vi "MainPanel_20170525.vi"() -> (0 "ErrorOut":errorcluster)   [LabVIEW 2018] (continued)
-inf, -inf, -inf, -inf, -inf, -inf, -inf, -inf, -inf, -inf, -inf, -inf, -inf, -inf, -inf, -inf, -inf, -inf, -inf, -inf, -inf, -inf, -inf, -inf, -inf, -inf, -inf, -inf, -inf, -inf, -inf, -inf, -inf, -inf, -inf, -inf, -inf, -inf, -inf, -inf, -inf, -inf, -inf, -inf, -inf, -inf, -inf, -inf, -inf, -inf, -inf, -inf, -inf, -inf, -inf, -inf, -inf, -inf, -inf, -inf, -inf, -inf, -inf, -inf, -inf, -inf, -inf, -inf, -inf, -inf, -inf, -inf, -inf, -inf, -inf, -inf, -inf, -inf, -inf, -inf, -inf, -inf, -inf, -inf, -inf, -inf, -inf, -inf, -inf, -inf, -inf, -inf, -inf, -inf, -inf, -inf, -inf, -inf, -inf, -inf, -inf, -inf, -inf, -inf, -inf, -inf, -inf, -inf, -inf, -inf, -inf, -inf, -inf, -inf, -inf, -inf, -inf, -inf, -inf, -inf, -inf, -inf, -inf, -inf, -inf, -inf, -inf, -inf, -inf, -inf, -inf, -inf, -inf, -inf, -inf, -inf, -inf, -inf, -inf, -inf, -inf, -inf, -inf, -inf, -inf, -inf, -inf, -inf, -inf, -inf, -inf, -inf, -inf, -inf, -inf, -inf, -inf, -inf, -inf, -inf, -inf, -inf, -inf, -inf, -inf, -inf, -inf, -inf, -inf, -inf, -inf, -inf, -inf, -inf, -inf, -inf, -inf, -inf, -inf, -inf, -inf, -inf, -inf, -inf, -inf, -inf, -inf, -inf, -inf, -inf, -inf, -inf, -inf, -inf, -inf, -inf, -inf, -inf, -inf, -inf, -inf, -inf, -inf, -inf, -inf, -inf, -inf, -inf, -inf, -inf, -inf, -inf, -inf, -inf, -inf, -inf, -inf, -inf, -inf, -inf, -inf, -inf, -inf, -inf, -inf, -inf, -inf, -inf, -inf, -inf, -inf, -inf, -inf, -inf, -inf, -inf, -inf, -inf, -inf, -inf, -inf, -inf, -inf, -inf, -inf, -inf, -inf, -inf, -inf, -inf, -inf, -inf, -inf, -inf, -inf, -inf, -inf, -inf, -inf, -inf, -inf, -inf, -inf, -inf, -inf, -inf, -inf, -inf, -inf, -inf, -inf, -inf, -inf, -inf, -inf, -inf, -inf, -inf, -inf, -inf, -inf, -inf, -inf, -inf, -inf, -inf, -inf, -inf, -inf, -inf, -inf, -inf, -inf, -inf, -inf, -inf, -inf, -inf, -inf, -inf, -inf, -inf, -inf, -inf, -inf, -inf, -inf, -inf, -inf, -inf, -inf, -inf, -inf, -inf, -inf, -inf, -inf, -inf, -inf, -inf, -inf, -inf, -inf, -inf, -inf, -inf, -inf, -inf, -inf, -inf, -inf, -inf, -inf, -inf, -inf, -inf, -inf, -inf, -inf, -inf, -inf, -inf, -inf, -inf, -inf, -inf, -inf, -inf, -inf, -inf, -inf, -inf, -inf, -inf, -inf, -inf, -inf, -inf, -inf, -inf, -inf, -inf, -inf, -inf, -inf, -inf, -inf, -inf, -inf, -inf, -inf, -inf, -inf, -inf, -inf, -inf, -inf, -inf, -inf, -inf, -inf, -inf, -inf, -inf, -inf, -inf, -inf, -inf, -inf, -inf, -inf, -inf, -inf, -inf, -inf, -inf, -inf, -inf, -inf, -inf, -inf, -inf, -inf, -inf, -inf, -inf, -inf, -inf, -inf, -inf, -inf, -inf, -inf, -inf, -inf, -inf, -inf, -inf, -inf, -inf, -inf, -inf, -inf, -inf, -inf, -inf, -inf, -inf, -inf, -inf, -inf, -inf, -inf, -inf, -inf, -inf, -inf, -inf, -inf, -inf, -inf, -inf, -inf, -inf, -inf, -inf, -inf, -inf, -inf, -inf, -inf, -inf, -inf, -inf, -inf, -inf, -inf, -inf, -inf, -inf, -inf, -inf, -inf, -inf, -inf, -inf, -inf, -inf, -inf, -inf, -inf, -inf, -inf, -inf, -inf, -inf, -inf, -inf, -inf, -inf, -inf, -inf, -inf, -inf, -inf, -inf, -inf, -inf, -inf, -inf, -inf, -inf, -inf, -inf, -inf, -inf, -inf, -inf, -inf, -inf, -inf, -inf, -inf, -inf, -inf, -inf, -inf, -inf, -inf, -inf, -inf, -inf, -inf, -inf, -inf, -inf, -inf, -inf, -inf, -inf, -inf, -inf, -inf, -inf, -inf, -inf, -inf, -inf, -inf, -inf, -inf, -inf, -inf, -inf, -inf, -inf, -inf, -inf, -inf, -inf, -inf, -inf, -inf, -inf, -inf, -inf, -inf, -inf, -inf, -inf, -inf, -inf, -inf, -inf, -inf, -inf, -inf, -inf, -inf, -inf, -inf, -inf, -inf, -inf, -inf, -inf, -inf, -inf, -inf, -inf, -inf, -inf, -inf, -inf, -inf, -inf, -inf, -inf, -inf, -inf, -inf, -inf, -inf, -inf, -inf, -inf, -inf, -inf, -inf, -inf, -inf, -inf, -inf, -inf, -inf, -inf, -inf, -inf, -inf, -inf, -inf, -inf, -inf, -inf, -inf, -inf, -inf, -inf, -inf, -inf, -inf, -inf, -inf, -inf, -inf, -inf, -inf, -inf, -inf, -inf, -inf, -inf, -inf, -inf, -inf, -inf, -inf, -inf, -inf, -inf, -inf, -inf, -inf, -inf, -inf, -inf, -inf, -inf, -inf, -inf, -inf, -inf, -inf, -inf, -inf, -inf, -inf, -inf, -inf, -inf, -inf, -inf, -inf, -inf, -inf, -inf, -inf, -inf, -inf, -inf, -inf, -inf, -inf, -inf, -inf, -inf, -inf, -inf, -inf, -inf, -inf, -inf, -inf, -inf, -inf, -inf, -inf, -inf, -inf, -inf, -inf, -inf, -inf, -inf, -inf, -inf, -inf, -inf, -inf, -inf, -inf, -inf, -inf, -inf, -inf, -inf, -inf, -inf, -inf, -inf, -inf, -inf, -inf, -inf, -inf, -inf, -inf, -inf, -inf, -inf, -inf, -inf, -inf, -inf, -inf, -inf, -inf, -inf, -inf, -inf, -inf, -inf, -inf, -inf, -inf, -inf, -inf, -inf, -inf, -inf, -inf, -inf, -inf, -inf, -inf, -inf, -inf, -inf, -inf, -inf, -inf, -inf, -inf, -inf, -inf, -inf, -inf, -inf, -inf, -inf, -inf, -inf, -inf, -inf, -inf, -inf, -inf, -inf, -inf, -inf, -inf, -inf, -inf, -inf, -inf, -inf, -inf, -inf]
  out "df (Hz)":dbl=15258.7890625
  in  "AutoScale Y Noise":bool caption="AutoScale Y"
  in  "AvgAvg":bool caption="Average over 1 minute"
  out "Freq History 72 Co":cluster{dbl, dbl, dbl}(graph)
  out "Freq History 84 Co":cluster{dbl, dbl, dbl}(graph)
  out "84CoCalFrq":dbl format="%#.9f"
  out "MaxValue_Cal_84X":dbl format="%#.2g"
  out "84CoBeacFrq":dbl format="%#.9f"
  out "MaxValue_Cal_72X":dbl format="%#.2g"
  out "72CoCalFrq":dbl format="%#.9f"
  out "72CoBeacFrq":dbl format="%#.2f"
  out "ADAM-Noise":dbl format="%#.2g"
  out "ADAM-CalEncl":dbl format="%#.2g"
  out "ADAM-XPol":dbl format="%#.2g"
  out "ADAM-Co":dbl format="%#.2g"
  out "TE_Front":dbl format="%#.2g"
  out "TE_Bottom":dbl format="%#.2g"
  out "TE_Air":dbl format="%#.2g"
  out "InclEl":dbl format="%#.2g"
  out "InclAz":dbl format="%#.2g"
  out "MaxValue_Cal_84Co":dbl format="%#.2g"
  out "MaxValue_Cal_72Co":dbl format="%#.2g"
  out "+28":dbl format="%#.2g"
  out "+15":dbl format="%#.2g"
  out "+12":dbl format="%#.2g"
  out "+6":dbl format="%#.2g"
  out "+5":dbl format="%#.2g"
  out "-5V":dbl format="%#.2g"
  out "ConnextIntTemp":dbl format="%#.2g"
  in  "AlarmThresholds_OneChan":T12={"Enbl"=FALSE, "ErrsAndWarns"={2.256637168141593, 5.663716814159292, 7.168141592920354, 9.336283185840708}} {"ErrsAndWarns" scale=0.0..10.0}
  in  "AlarmSettings":T13={"TC13"={"Enbl"=FALSE, "ErrsAndWarns"={0.0, 5.663716814159292, 7.168141592920354, 8.584070796460177}}, "AI1"={"Enbl"=FALSE, "ErrsAndWarns"={0.0, 5.663716814159292, 7.168141592920354, 8.584070796460177}}, "AI2"={"Enbl"=FALSE, "ErrsAndWarns"={0.0, 5.663716814159292, 7.168141592920354, 8.584070796460177}}, "AI3"={"Enbl"=FALSE, "ErrsAndWarns"={0.0, 5.663716814159292, 7.168141592920354, 8.584070796460177}}, "AI4"={"Enbl"=FALSE, "ErrsAndWarns"={0.0, 5.663716814159292, 7.168141592920354, 8.584070796460177}}, "AI5"={"Enbl"=FALSE, "ErrsAndWarns"={0.0, 5.663716814159292, 7.168141592920354, 8.584070796460177}}, "AI6"={"Enbl"=FALSE, "ErrsAndWarns"={0.0, 5.663716814159292, 7.168141592920354, 8.584070796460177}}, "AI18"={"Enbl"=FALSE, "ErrsAndWarns"={0.0, 5.663716814159292, 7.168141592920354, 8.584070796460177}}, "AI19"={"Enbl"=FALSE, "ErrsAndWarns"={0.0, 5.663716814159292, 7.168141592920354, 8.584070796460177}}, "TE1"={"Enbl"=FALSE, "ErrsAndWarns"={0.0, 5.663716814159292, 7.168141592920354, 8.584070796460177}}, "TE2"={"Enbl"=TRUE, "ErrsAndWarns"={0.0, 5.663716814159292, 7.168141592920354, 8.584070796460177}}, "TE3"={"Enbl"=FALSE, "ErrsAndWarns"={0.0, 5.663716814159292, 7.168141592920354, 8.584070796460177}}, "ADAM1"={"Enbl"=FALSE, "ErrsAndWarns"={0.0, 5.663716814159292, 7.168141592920354, 8.584070796460177}}, "ADAM2"={"Enbl"=FALSE, "ErrsAndWarns"={0.0, 5.663716814159292, 7.168141592920354, 8.584070796460177}}, "ADAM3"={"Enbl"=FALSE, "ErrsAndWarns"={0.0, 5.663716814159292, 7.168141592920354, 8.584070796460177}}, "ADAM4"={"Enbl"=FALSE, "ErrsAndWarns"={0.0, 5.663716814159292, 7.168141592920354, 8.584070796460177}}, "72CoBeacFreq"={"Enbl"=FALSE, "ErrsAndWarns"={0.0, 5.663716814159292, 7.168141592920354, 8.584070796460177}}, "72CoCalFreq"={"Enbl"=FALSE, "ErrsAndWarns"={0.0, 5.663716814159292, 7.168141592920354, 8.584070796460177}}, "84CoBeacFreq"={"Enbl"=FALSE, "ErrsAndWarns"={0.0, 5.663716814159292, 7.168141592920354, 8.584070796460177}}, "84CoCalFreq"={"Enbl"=FALSE, "ErrsAndWarns"={0.0, 5.663716814159292, 7.168141592920354, 8.584070796460177}}, "72Co_CalTonePwr"={"Enbl"=FALSE, "ErrsAndWarns"={-110.0, -90.0, -65.0, -60.0}}, "72X_CalTonePwr"={"Enbl"=FALSE, "ErrsAndWarns"={0.0, 5.663716814159292, 7.168141592920354, 8.584070796460177}}, "84Co_CalTonePwr"={"Enbl"=FALSE, "ErrsAndWarns"={0.0, 5.663716814159292, 7.168141592920354, 8.584070796460177}}, "84X_CalTonePwr"={"Enbl"=FALSE, "ErrsAndWarns"={0.0, 5.663716814159292, 7.168141592920354, 8.584070796460177}}} {"84X_CalTonePwr"."ErrsAndWarns" scale=-120.0..-45.0; "72X_CalTonePwr"."ErrsAndWarns" scale=-120.0..-45.0; "84Co_CalTonePwr"."ErrsAndWarns" scale=-120.0..-45.0; "72Co_CalTonePwr"."ErrsAndWarns" scale=-120.0..-45.0; "84CoCalFreq"."ErrsAndWarns" scale=24.9..25.1; "84CoBeacFreq"."ErrsAndWarns" scale=25.5..27.0; "72CoCalFreq"."ErrsAndWarns" scale=24.9..25.1; "72CoBeacFreq"."ErrsAndWarns" scale=25.5..27.0; "ADAM4"."ErrsAndWarns" scale=30.0..52.0; "ADAM3"."ErrsAndWarns" scale=30.0..52.0; "ADAM2"."ErrsAndWarns" scale=30.0..52.0; "ADAM1"."ErrsAndWarns" scale=30.0..52.0; "TE3"."ErrsAndWarns" scale=30.0..52.0; "TE2"."ErrsAndWarns" scale=30.0..52.0; "TE1"."ErrsAndWarns" scale=20.0..52.0; "AI19"."ErrsAndWarns" scale=0.0..60.0; "AI18"."ErrsAndWarns" scale=-10.0..10.0; "AI6"."ErrsAndWarns" scale=0.0..35.0; "AI5"."ErrsAndWarns" scale=0.0..20.0; "AI4"."ErrsAndWarns" scale=0.0..15.0; "AI3"."ErrsAndWarns" scale=0.0..10.0; "AI2"."ErrsAndWarns" scale=0.0..10.0; "TC13"."ErrsAndWarns" scale=-10.0..40.0}
  out "Elapsed_SNR_Timer":dbl caption="Elapsed SNR Timer"
  out "BlowerPower":dbl format="%#.2g"
  out "GeneratorExhaust":dbl format="%#.2g"
  in  "Trouble Shooting Tabs":T14(tab)
  out "Q Probes":T15
  out "Probe 21":fxp<+/-,24,5>=-4.57763671875e-05
  out "Probe 22":fxp<+/-,54,35>=-15871.999969482422
  out "Probe 23":fxp<+/-,54,1>=-7.629394517039145e-06
  out "Probe 24":fxp<+/-,16,1>
  out "I Probes":T15
  out "Probe 3":fxp<+/-,39,24>=-0.003662109375
  out "Probe 1":i16=-27
  out "Probe 2":fxp<+/-,16,16>
  out "Probe 5":fxp<+/-,16,2>
  out "Probe 7":fxp<+/-,18,1>
  out "Probe Offsetd":fxp<+/-,16,16>
  in  "Target to Probe":T16=enum."4"
  in  "Time Domain Tabs":enum32{"72 Co", "72 X", "84 Co", "84 X"}(tab)
  out "TimeDomainCal 72Co":ext[](graph)
  out "TimeDomainBeac 72Co":ext[](graph)
  out "TimeDomainCal 72 X":ext[](graph)
  out "TimeDomainBeacon 72 X":ext[](graph)
  out "TimeDomainCal 84 Co":ext[](graph)
  out "TimeDomain Beac 84 Co":ext[](graph)
  out "TimeDomainCal 84 X":ext[](graph)
  out "TimeDomainBeacon 84 X":ext[](graph)
  out "Memory Used":dbl(graph)=797012.0
  out "CalShift 2":dbl=24999500.0 format="%#_10g"
  out "BeaconShift 2":dbl=26246000.0 format="%#_10g"
  out "BeaconShift":dbl=26246000.0 format="%#_10g"
  out "CalShift":dbl=24999500.0 format="%#_10g"
  out "Memory Used By LV (KB)":dbl=797012.0
  out "BeaconShift 4":dbl=26244800.0 format="%#_10g"
  out "BeaconShift 3":dbl=26246000.0 format="%#_10g"
  out "CalShift 3":dbl=24999500.0 format="%#_10g"
  out "CalShift 4":dbl=24998000.0 format="%#_10g"
  in  "MemoryPlotRate":dbl=30.0 format="%#_13g"
  out "SPVSR_Count":i32
  out "SPVSR_Queue":i32
  out "FP_Count":i32
  out "# in FP queue":i32
  out "Digitizer 1 Init Attempts":i32
  out "Digitizer 2 Init Attempts":i32
  in  "noise_ctrl":bool
  in  "72GHz_ctrl":bool=TRUE
  in  "84GHz_ctrl":bool=TRUE
  in  "base path":path=path "C:/ConnexTest" caption="Local Storage path for data logs"
  in  "NAS path":path=path "C:/ConnexData"
  in  "ThreshFile":path=path "C:/Users/bruce wayne/Desktop/ATA_Source_20180912/thresholds.csv" caption="Thresholds file"
  in  "Exit":bool
  in  "Stop":bool
  # "Ver 20220331"
  # "Low pass filter applied to chart.\nTo turn filter off, set New Value Weighting to 1."
  # "Angle_out = [(V_reading – Vmin) / Vmax ) * (Angle_max - Angle_min) + Angle_min + Angle_offset ] * (-1 if pos_neg toggle switch is on)\n\nThe default (equivalent to current equation) values would be\nVmin = 0\nVmax = 4.5\nAngle_min = -90\nAngle_range = Angle_max-Angle_min\nAngle_max = 90\nAngle_offset = 0\nPos_neg = off"
  # "v 2022_03_08"
  # "72 Cross Tracking Frequency is linked to 72 Co"
  # "84 Cross Tracking Frequency is linked to 84 Co"
  # "72 GHz"
  # "84 GHz"
  # "Do not use \"Tab\" to commit values. Use \"Enter\" or click off of the control."
  # "Enable/disable"
  # "The digital readouts display the same errors and \nwarnings with more precision."
  # "Low Error"
  # "Low Warning"
  # "High Warning"
  # "High Error"
  # "seconds"
  # "Copyright © 2022 Epimedia, Inc. All Rights Reserved.\n\nThe Epimedia Application Library is Copyright © 2009-2022 Epimedia, Inc. \nAll Rights Reserved. Used under license."
  # "I Probes"
  # "Q Probes"
  # "-1 to 0.999, d:7.629e-6"
  # "Shifted"
  # "I16"
  # "-1 to 1, d:1.92e-7"
  # "From digitizer"
  # "Filtered Step 4"
  # "-3.27e4 to 3.27e4, d:1"
  # "-1 to 1, d:1.92e-7"
  # "To FXP"
  # "Scaled and reduced data size"
  # "-3.27e4 to 3.27e4, d:1"
  # "-1 to 1, d:1.92e-7"
  # "Filtered Step 5"
  # "-6.55e4 to 6.55e4, d:3.05e-5"
  # "-8.39e6 to 8.39e6, d:1.19e-7"
  # "Scaled"
  # "Scaled after Step 5"
  # "XXX"
  # "-2 to 2, d:2.38e-7"
  # "-2 to 1.999, d:6.10e-5"
  # "Filtered Step 6"
  # "Filtered stage A"
  # "-1.677e7 to 1.677e7, d:2.38e-7"
  # "Scaled after Step 6"
  # "XXX"
  # "-2.62e5 to 2.62e5, d:6.10e-5"
  # "Scaled (Step 1 Scale)"
  # "-1 to 1, d:1.82e-12"
  # "Filtered Step 7"
  # "-8.39e6 to 8.39e6, d:1.82e-12"
  # "Filtered after Step 7"
  # "XXX"
  # "-8.39e6 to 8.39e6, d:1.82e-12"
  # "Sent to host\nIdentical to 18"
  # "Noise Floor"
  # "-4 to 4"
  # "-3.35e7 to 3.35e7, d:4.7e-7"
  # "-1 to 1, d:1.4e-14"
  # "-1 to .99, d:3.05e-5"
  # "The following shift variables are used to scale\nthe x-axis of the plots on the the Spectrum tab"
  # "The noise source has been disconnected. Please see technical manual for further information."
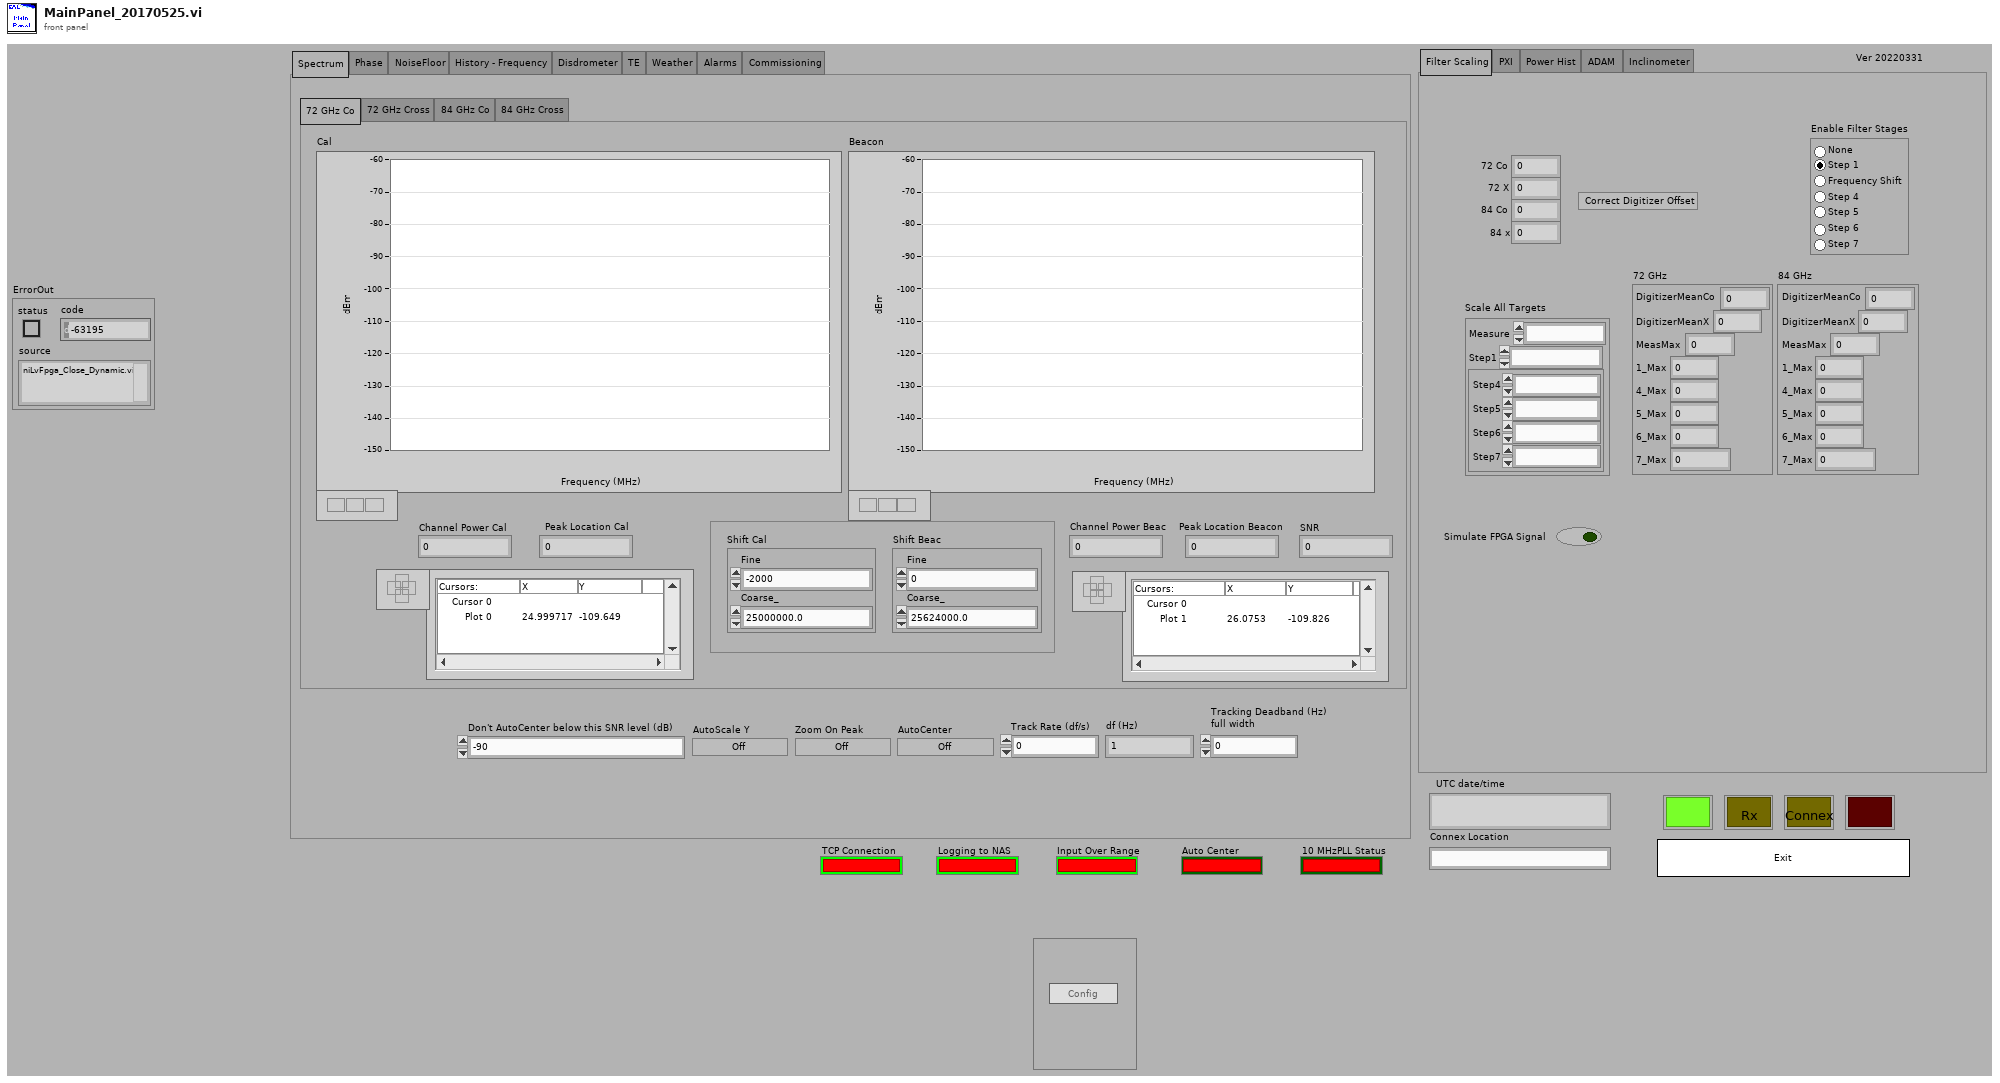
[diagram p1: front panel]
types:
  T1 = enum32{"Filter Scaling", "PXI", "Power Hist", "ADAM", "Inclinometer"}
  T2 = typedef "SaturationMonitor.ctl" = cluster{"MeasMean0":dbl, "MeasMean1":dbl, "MeasMax":dbl, "1_Max":dbl, "4_Max":dbl, "5_Max":dbl, "6_Max":dbl, "7_Max":dbl}
  T3 = typedef "ScaleTargetClust.ctl" = cluster{"Measure":fxp<+/-,16,1>, "Step1":fxp<+/-,17,17>, "Scale":T4}
  T4 = typedef "FPGA_Scale.ctl" = cluster{"Step4":fxp<+/-,23,23>, "Step5":fxp<+/-,23,23>, "Step6":fxp<+/-,23,23>, "Step7":fxp<+/-,23,23>}
  T5 = typedef "FilterEnableRadio.ctl" = enum32{"None", "Step 1", "Frequency Shift", "Step 4", "Step 5", "Step 6", "Step 7"}
  T6 = cluster{"Cal Smooth":dbl, "Beac Smooth":dbl, "Cal Smooth":dbl, "Beac Smooth":dbl, "Cal Smooth":dbl, "Beac Smooth":dbl, "Cal Smooth":dbl, "Beac Smooth":dbl}
  T7 = typedef "Inclinometer_User_Cfg.ctl" = cluster{"Vmin":dbl, "Vmax":dbl, "Angle_min":dbl, "Angle_max":dbl, "Offset":dbl, "Pos_Neg":bool}
  T8 = cluster{"Ai18_InclinometerAz":dbl, "Ai19_InclinometerEl":dbl}
  T9 = enum32{"Spectrum", "Phase", "NoiseFloor", "History - Frequency", "Disdrometer", "TE", "Weather", "Alarms", "Commissioning"}
  T10 = enum32{"72 GHz Co", "72 GHz Cross", "84 GHz Co", "84 GHz Cross"}
  T11 = typedef "FreqShift.ctl" = cluster{"Fine":dbl, "Coarse_":dbl}
  T12 = typedef "AlarmThresh_OneChan.ctl" = cluster{"Enbl":bool, "ErrsAndWarns":cluster{dbl, dbl, dbl, dbl}}
  T13 = typedef "AlarmSettingsClust.ctl" = cluster{"TC13":T12, "AI1":T12, "AI2":T12, "AI3":T12, "AI4":T12, "AI5":T12, "AI6":T12, "AI18":T12, "AI19":T12, "TE1":T12, "TE2":T12, "TE3":T12, "ADAM1":T12, "ADAM2":T12, "ADAM3":T12, "ADAM4":T12, "72CoBeacFreq":T12, "72CoCalFreq":T12, "84CoBeacFreq":T12, "84CoCalFreq":T12, "72Co_CalTonePwr":T12, "72X_CalTonePwr":T12, "84Co_CalTonePwr":T12, "84X_CalTonePwr":T12}
  T14 = enum32{"FPGA Probes", "Time Domain", "Win Probes", "Cal Tone Controls", "Paths"}
  T15 = cluster{"Probe 8":fxp<+/-,18,1>, "Probe 9":fxp<+/-,24,1>, "Probe 10":fxp<+/-,24,1>, "Probe 11":fxp<+/-,24,1>, "Probe 12":fxp<+/-,47,24>, "Probe 13":fxp<+/-,24,1>, "Probe 14":fxp<+/-,25,2>, "Probe 15":fxp<+/-,48,25>, "Probe 16":fxp<+/-,24,1>, "Probe 17":fxp<+/-,25,2>, "Probe 18":fxp<+/-,48,25>, "Probe 19":fxp<+/-,24,1>, "Probe20":fxp<+/-,24,1>}
  T16 = typedef "TargetNumber.ctl" = enum16{"1", "2", "3", "4"}
  T17 = typedef "LogLoopEnum.ctl" = enum16{"Log_Init", "Log_Config", "Log_CfgAlarm", "Log_TimeDomain", "Log_Tone", "Log_NoiseTrace", "Log_NoiseSum", "Log_DO", "Log_AI", "Log_TC", "Log_Disdrom", "Log_Weather", "Log_TE", "Log_ADAM", "Log_UPS", "Log_ChkTime", "Log_Alarm", "Log_SSH", "Log_Write", "Log_Exit"}
  T18 = typedef "TCP_Loop.ctl" = enum16{"TCP_Write", "TCP_ChkTime", "TCP_Exit"}
  T19 = typedef "10Hz_Loop_Enum.ctl" = enum16{"10Hz_Init", "10Hz_Cfg", "10Hz_NewData", "10Hz_Write", "10Hz_Stop"}
  T20 = typedef "FP_Loop_Clust.ctl" = cluster{"Alarms":T21, "Spectrum 1":dbl[], "Spectrum 2":dbl[], "Spectrum 3":dbl[], "Spectrum 4":dbl[], "HistoryWeighting":dbl, "NoiseFloorSums":T22, "PwrHist":T23}
  T21 = typedef "DigOutClust.ctl" = cluster{"Green":bool, "Rx_Yell":bool, "Cx_Yell":bool, "Red":bool, "Source":string}
  T22 = typedef "NoiseFLoorSums.ctl" = cluster{"1":dbl, "2":dbl, "3":dbl, "4":dbl}
  T23 = typedef "PowerHistory_All.ctl" = cluster{"72Co":cluster{"Cal":dbl, "Cal Smooth":dbl, "Beac":dbl, "Beac Smooth":dbl, "NoiseFloorSum":dbl, "NoiseFloorSum Smooth":dbl}, "72X":cluster{"Cal":dbl, "Cal Smooth":dbl, "Beac":dbl, "Beac Smooth":dbl, "NoiseFloorSum":dbl, "NoiseFloorSum Smooth":dbl}, "84Co":cluster{"Cal":dbl, "Cal Smooth":dbl, "Beac":dbl, "Beac Smooth":dbl, "NoiseFloorSum":dbl, "NoiseFloorSum Smooth":dbl}, "84X":cluster{"Cal":dbl, "Cal Smooth":dbl, "Beac":dbl, "Beac Smooth":dbl, "NoiseFloorSum":dbl, "NoiseFloorSum Smooth":dbl}}
  T24 = typedef "AI_Type_Enum.ctl" = enum16{"AI", "TC"}
  T25 = typedef "HWQueueElements.ctl" = enum16{"HW_Init", "HW_UpdtCfg", "HW_Start", "HW_Pause", "HW_Run", "HW_Cls", "HW_Exit"}
  T26 = typedef "FP_Loop_Enum.ctl" = enum16{"FP_Init", "FP_Scale", "FP_Tone", "FP_Noise", "FP_Probes", "FP_PXI", "FP_AI", "FP_TC", "FP_PWR_Hist", "FP_Alarm", "FP_Exit"}
  T27 = typedef "DigiLoopEnum.ctl" = enum16{"Dig_Init", "Digi_Write", "Digi_Exit"}
  T28 = typedef "NoiseQueueElements.ctl" = enum16{"Noise_Startup", "Noise_Init", "Noise_Macro", "Noise_Config", "Noise_NewData", "Noise_Transform", "Noise_SumdTrace", "Noise_Send", "Noise_Probes", "Noise_Exit"}
  T29 = typedef "MasterCluster.ctl" = cluster{"Admin":T30, "RTConfig":T32, "SMS":T33, "FPGA":T34, "Config":T35, "Stat":T41, "Alarm":T13}
  T30 = typedef "AdminCluster.ctl" = cluster{"Lvl":T31, "Pwd":string}
  T31 = typedef "UserLevelEnum.ctl" = enum16{"Admin", "Operator"}
  T32 = typedef "RT_Config.ctl" = cluster{"Arm":bool, "Number":dbl, "String":string}
  T33 = typedef "SMSDataCluster.ctl" = cluster{"Enbl?":bool, "Addr":string[]}
  T34 = typedef "FPGA_Config_Clust.ctl" = cluster{"Target":T16, "Channel":T16, "Ref1":refnum<k20>, "Ref2":refnum<k20>}
  T35 = typedef "Config_Clust.ctl" = cluster{"UsrCfg":T36, "FP_User":T38}
  T36 = typedef "UserConfig.ctl" = cluster{"Paths":T37, "SampleRate":dbl}
  T37 = typedef "PathsCluster.ctl" = cluster{"CfgFile":path, "LogFolder":path, "LogFile":path, "NAS path":path, "ThreshFile":path, "RedunFolder":path}
  T38 = typedef "FrontPanel_UserConfig.ctl" = cluster{"#NoiseSums":u32, "Max_df":u32, "AvgAvg":bool, "#Avg":u16, "AutoCenter":bool, "Inclin":T7, "1":T39, "2":T39, "3":T39, "4":T39, "Target to Probe":T16, "SNR_Thresh":dbl, "Paths":T37, "Connex_Location":string, "SimulateFPGA":bool, "Deadband":dbl}
  T39 = typedef "FP_UserTargetConfig.ctl" = cluster{"Cal_":T11, "Beac":T11, "Scale":T4, "Offset":fxp<+/-,16,16>, "Scale_Noise":fxp<+/-,30,30>, "Scale_Step1":fxp<+/-,17,17>, "Scale_In_RT":ext, "ScaleMeas":fxp<+/-,16,1>, "FreqsToRemove":i32[], "Width":i32[], "ScaleMeasEnum":T40, "FilterEnab":T5}
  T40 = typedef "ScaleMeasure.ctl" = enum16{"1", "10", "50", "42"}
  T41 = typedef "SystemStatusCluster.ctl" = cluster{"SysState":T42, "TrackRate":bool, "AutoCentr":bool}
  T42 = typedef "SystemStateEnum.ctl" = enum16{"Init", "Idle", "Running", "System Fault", "System Error", "Exit"}
  T43 = typedef "DataQueueElements.ctl" = enum16{"Data_Init", "Data_Config", "Data_AddData", "Data_FreqShift", "Data_FPGA_Write", "Data_Transform", "Data_Send", "Data_Exit"}
  T44 = typedef "MainQueueElements.ctl" = enum16{"Spvsr_InitQ", "Spvsr_RfrshPnl", "Spvsr_InitSW", "Spvsr_InitCtrls", "Spvsr_Cursors", "Spvsr_StrtHWLp", "Spvsr_Stop", "Spvsr_NewData", "Spvsr_ScaleGraphs", "Spvsr_Error", "Spvsr_About", "Spvsr_Config", "Spvsr_FPConfig", "Spvsr_AlarmCfg", "Spvsr_DigitzOffs", "FP_AO_ctrl", "Spvsr_RestartWarn", "Spvsr_AutoCenter", "Spvsr_TrackRate", "Spvsr_ChkTime", "Spvsr_Admin", "Spvsr_Exit"}
  T45 = typedef "HDF5_10HzRefs.ctl" = cluster{"72Co_dset":T46, "84Co_dset":T46, "FileRef":T46}
  T46 = typedef "hid_t.ctl" = i32
  T47 = typedef "WatchdogTimer_Enum.ctl" = enum16{"ResetAll", "CheckAll", "HW1", "HW2", "Tones", "FP", "Noise", "Log", "TCP", "AI", "TC", "ADAM", "Disdrom", "TE", "Weather"}
  T48 = enum8{"Enabled", "Disabled", "Disabled and Grayed Out"}
  T49 = typedef "AI_Loop_Enum.ctl" = enum16{"AI_Init", "AI_Config", "AI_Alarm", "AI_Read", "AI_ChkTime", "AI_Exit"}
  T50 = typedef "LVCursorListTypeDef.ctl" = cluster{"Name":string, "Color":u32, "Style":u8, "Point Style":u8, "Name Visible":bool, "Allow Drag":bool, "Cursor Mode":u32, "Plot":i32, "Index":i32, "Position":cluster{"X":dbl, "Y":dbl}, "X Scale":u32, "Y Scale":u32, "Watch Plots":i32[], "Watch All Plots":bool, "Plot Area":i32, "Label Offset":cluster{"X":dbl, "Y":dbl}}[]
  T51 = typedef "AO_Loop_Enum.ctl" = enum16{"AO_Init", "AO_Write", "AO_Exit"}
  T52 = typedef "TargetToneData.ctl" = cluster{"Cal":T53, "Beac":T53, "Time":timestamp[], "Saturat":T2}
  T53 = typedef "ChannelToneData.ctl" = cluster{"Shift_":dbl, "Peak_ToFPGA":dbl, "MaxValue":dbl, "MaxIndex":i32, "Tone":T54, "TimeDomainI":ext[], "TimeDomainQ":ext[], "PwrSpectrum":dbl[], "RunningAvgFreq":dbl, "ISpectPos":dbl[], "ISpectNeg":dbl[], "QSpectPos":dbl[], "QSpectNeg":dbl[], "10Hz_PwrSpectr":dbl[][], "SNR":dbl, "AliasWarn":bool, "10Hz_Peak":dbl[], "ISpect+-":dbl[], "QSpect+-":dbl[], "TimeStamp":timestamp, "I_Index":ext[], "Q_Index":ext[], "10MHz":bool}
  T54 = typedef "ToneInfoClust.ctl" = cluster{"PkLocTrak":dbl, "PkLocDisp":dbl, "df_":dbl, "ZoomPwr":dbl[], "Phase":dbl, "PhaseOld":dbl, "AboveThresh?":bool, "MaxI":dbl, "MaxQ":dbl, "median":dbl, "ISpect":dbl[], "QSpect":dbl[], "DeltaPhase":dbl}
  T55 = typedef "NoiseFloorData.ctl" = cluster{"df":dbl, "AvgAvgSpectrum":dbl[], "FFT_Index":i32[], "Avg'd":dbl[], "Sum":dbl, "SumdSpectrum":dbl[], "SumCount":u32, "DayOfYear":i32}
  T56 = typedef "FPGA_Probes.ctl" = cluster{"Probe 1":i16, "Probe 2":fxp<+/-,16,16>, "Probe 3":fxp<+/-,39,24>, "Probe 4":fxp<+/-,39,24>, "Probe 5":fxp<+/-,16,2>, "Probe 6":fxp<+/-,33,19>, "Probe 7":fxp<+/-,18,1>, "Probe 7_1":fxp<+/-,18,1>, "IProbe":cluster{"Probe 8":fxp<+/-,18,1>, "Probe 9":fxp<+/-,24,1>, "Probe 10":fxp<+/-,24,1>, "Probe 11":fxp<+/-,24,1>, "Probe 12":fxp<+/-,47,24>, "Probe 13":fxp<+/-,24,1>, "Probe 14":fxp<+/-,25,2>, "Probe 15":fxp<+/-,48,25>, "Probe 16":fxp<+/-,24,1>, "Probe 17":fxp<+/-,25,2>, "Probe 18":fxp<+/-,48,25>, "Probe 19":fxp<+/-,24,1>, "Probe20":fxp<+/-,24,1>}, "Probe 21":fxp<+/-,24,5>, "Probe 22":fxp<+/-,54,35>, "Probe 23":fxp<+/-,54,1>, "Probe 24":fxp<+/-,16,1>, "Probe Offsetd":fxp<+/-,16,16>, "CalShiftProbe":fxp<+/-,48,0>, "QProbe":cluster{"Probe 8":fxp<+/-,18,1>, "Probe 9":fxp<+/-,24,1>, "Probe 10":fxp<+/-,24,1>, "Probe 11":fxp<+/-,24,1>, "Probe 12":fxp<+/-,47,24>, "Probe 13":fxp<+/-,24,1>, "Probe 14":fxp<+/-,25,2>, "Probe 15":fxp<+/-,48,25>, "Probe 16":fxp<+/-,24,1>, "Probe 17":fxp<+/-,25,2>, "Probe 18":fxp<+/-,48,25>, "Probe 19":fxp<+/-,24,1>, "Probe20":fxp<+/-,24,1>}, "AI_Over":bool, "10MHzLocked":bool}
  T57 = typedef "PXI_Health.ctl" = cluster{"Temperatures":string[][], "Fans":string[][], "Voltages":string[][]}
  T58 = typedef "All_AI_Error_and_Data.ctl" = cluster{"AI":T59, "AllErrorStatus":T60}
  T59 = typedef "AI_Clust.ctl" = cluster{"TimeString":string, "Time Stamp":dbl, "AI0_Unused":dbl, "AI1_-5V":dbl, "AI2_+5V":dbl, "AI3_+6V":dbl, "AI4_+12V":dbl, "AI5_+15V":dbl, "AI6_+28V":dbl, "AI7_Unused":dbl, "Ai16_72GHz_CalPower":dbl, "Ai17_84GHz_CalPower":dbl, "Ai18_InclinAz":dbl, "Ai19_InclinEl":dbl, "Ai20_BlowerPwr":dbl, "Ai21_Unused":dbl, "Ai22_Unused":dbl, "Ai23_Unused":dbl, "InclinA_StdDev":dbl, "InclinB_StdDev":dbl, "InclinAz_Unfilt":dbl, "InclinEl_Unfilt":dbl}
  T60 = typedef "All_AI_Error_Status.ctl" = cluster{"AI 0":T61, "AI 1":T61, "AI 2":T61, "AI 3":T61, "AI 4":T61, "AI 5":T61, "AI 6":T61, "AI 7":T61, "AI 16":T61, "AI 17":T61, "AI 18":T61, "AI 19":T61, "AI 20":T61, "AI 21":T61, "AI 22":T61, "AI 23":T61}
  T61 = typedef "ErrorStatus.ctl" = cluster{"RX?":bool, "Warn":bool, "Error":bool, "Enabl":bool, "Source":string}
  T62 = typedef "All_TC_Error_and_Data.ctl" = cluster{"TCData":T63, "All_TC_ErrorStatus":T64}
  T63 = typedef "TC_Data_Structure.ctl" = cluster{"TimeStamp":dbl, "TimeString":string, "TC0_LP1_Hi":dbl, "TC1_LP1_MidHi":dbl, "TC2_LP1_Mid":dbl, "TC3_LP1_LoMid":dbl, "TC4_LP1_Lo":dbl, "TC5_LP2_Hi":dbl, "TC6_LP2_MidHi":dbl, "TC7_LP2_Mid":dbl, "TC8_LP2_LoMid":dbl, "TC9_LP2_Lo":dbl, "TC10_HVAC_Cond_In":dbl, "TC11_HVAC_Cond_Out":dbl, "TC12_Gen_Exhaust":dbl, "TC13_Amb_Inter":dbl, "TC14_Unused":dbl, "TC15_Unused":dbl, "TC16_Unused":dbl, "TC17_Unused":dbl, "TC18_Unused":dbl, "TC19_Unused":dbl, "TC20_Unused":dbl, "TC21_Unused":dbl, "TC22_Unused":dbl, "TC23_Unused":dbl, "TC24_Unused":dbl, "TC25_Unused":dbl, "TC26_Unused":dbl, "TC27_Unused":dbl, "TC28_Unused":dbl, "TC29_Unused":dbl, "TC30_Unused":dbl, "TC31_Unused":dbl}
  T64 = typedef "All_TC_Error_Status.ctl" = cluster{"TC 0":T61, "TC 1":T61, "TC 2":T61, "TC 3":T61, "TC 4":T61, "TC 5":T61, "TC 6":T61, "TC 7":T61, "TC 8":T61, "TC 9":T61, "TC 10":T61, "TC 11":T61, "TC 12":T61, "TC 13":T61, "TC 14":T61, "TC 15":T61, "TC 16":T61, "TC 17":T61, "TC 18":T61, "TC 19":T61, "TC 20":T61}
  T65 = typedef "AlarmDisplay.ctl" = cluster{"Alarms":T21, "SerialMeas":T66, "AllAlarms":T61[], "Elapsed_SNR_Timer":dbl, "Saturation":T67}
  T66 = typedef "SerialMeasurements_Clust.ctl" = cluster{"TE_Air":dbl, "TE_Bottom":dbl, "TE_Front":dbl, "ADAM-Co":dbl, "ADAM-XPol":dbl, "ADAM-CalEncl":dbl, "ADAM-Noise":dbl}
  T67 = typedef "Saturation_Status_Clust.ctl" = cluster{"84":bool[], "72":bool[]}
  T68 = cluster{"Cal":dbl, "Cal Smooth":dbl, "Beac":dbl, "Beac Smooth":dbl, "NoiseFloorSum":dbl, "NoiseFloorSum Smooth":dbl}
  T69 = typedef "Voltage_Display_Clust.ctl" = cluster{"AI0_Unused":dbl, "AI1_-5V":dbl, "AI2_+5V":dbl, "AI3_+6V":dbl, "AI4_+12V":dbl, "AI5_+15V":dbl, "AI6_+28V":dbl, "Ai16_72GHz_CalPower":dbl, "Ai17_84GHz_CalPower":dbl, "Ai18_InclinometerAz":dbl, "Ai19_InclinometerEl":dbl, "Az_StdDev":dbl, "El_StdDev":dbl, "Ai20_BlowerPower":dbl}
  T70 = typedef "TC_Display_Clust.ctl" = cluster{"TC0_LP1_Hi":dbl, "TC1_LP1_MidHi":dbl, "TC2_LP1_Mid":dbl, "TC3_LP1_LoMid":dbl, "TC4_LP1_Lo":dbl, "TC5_LP2_Hi":dbl, "TC6_LP2_MidHi":dbl, "TC7_LP2_Mid":dbl, "TC8_LP2_LoMid":dbl, "TC9_LP2_Lo":dbl, "TC10_HVAC_Cond_In":dbl, "TC11_HVAC_Cond_Out":dbl, "TC12_Gen_Exhaust":dbl, "TC13_Tamb_Interior":dbl}
  T71 = enum16{"Always On", "Always Off", "Off While Running"}
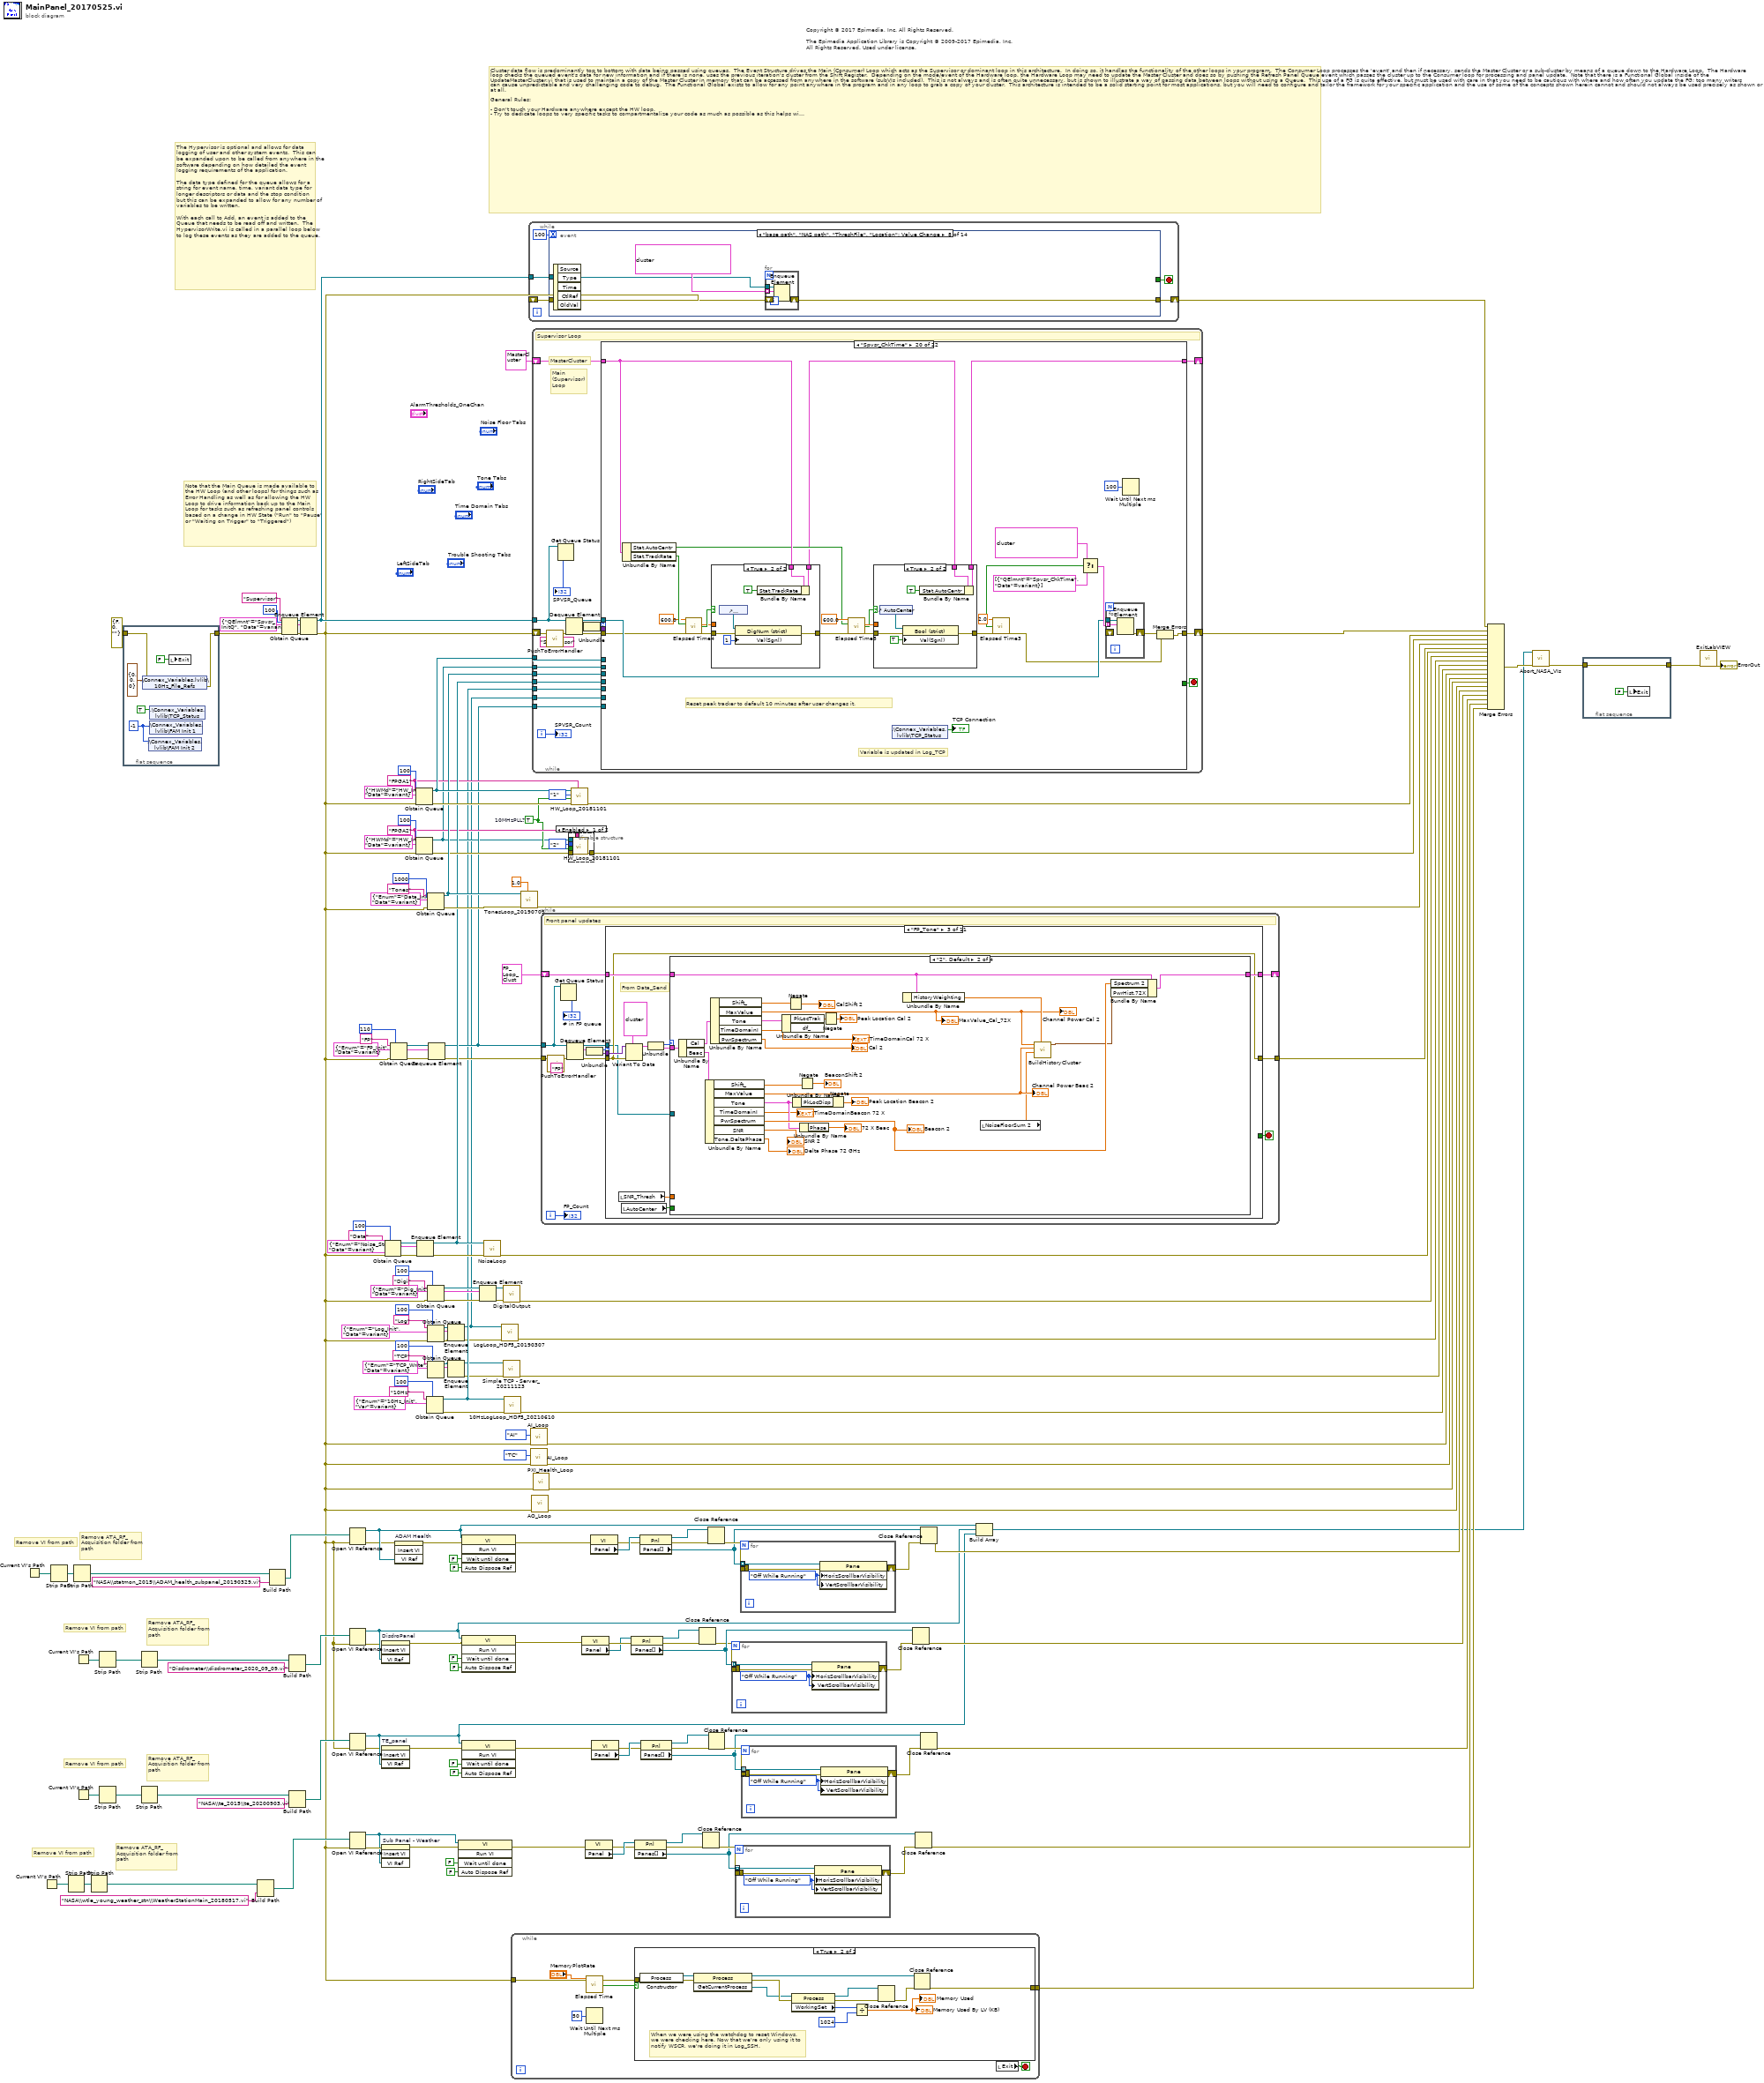
[diagram p0: block diagram]
diagram:
  w4 = cluster{"Enum":T17, "Data":variant} {"Enum"=enum."Log_Init", "Data"=variant} ("element")
  w7 = cluster{"Enum":T18, "Data":variant} {"Enum"=enum."TCP_Write", "Data"=variant}
  w75 = TRUE  # 10MHzPLL?
  w118 = "FPGA2" ("name (unnamed)")
  w99 = cluster{"Enum":T26, "Data":variant} {"Enum"=enum."FP_Init", "Data"=variant}
  w128 = cluster{"Enum":T27, "Data":variant} {"Enum"=enum."Dig_Init", "Data"=variant}
  w122 = cluster{"Enum":T28, "Data":variant} {"Enum"=enum."Noise_Startup", "Data"=variant}
  w119 = "FPGA1" ("name (unnamed)")
  w165 = cluster{"QElmnt":T44, "Data":variant} {"QElmnt"=enum."Spvsr_InitQ", "Data"=variant} ("Cluster")
  # "Remove ATA_RF_Acquisition folder from path"
  # "Remove VI from path"
  # "Remove ATA_RF_Acquisition folder from path"
  # "Remove VI from path"
  # "Remove ATA_RF_Acquisition folder from path"
  # "Remove VI from path"
  # "Remove ATA_RF_Acquisition folder from path"
  # "Remove VI from path"
  # "Note that the Main Queue is made available to the HW Loop (and other loops) for things such as Error Handling as well as for allowing the HW Loop to drive information back up to the Main Loop for tasks such as refreshing panel controls  based on a change in HW State (\"Run\" to \"Pause\" or \"Waiting on Trigger\" to \"Triggered\")"
  # "The Hypervisor is optional and allows for data logging of user and other system events.  This can be expanded upon to be called from anywhere in the software depending on how detailed the event logging requirements of the application.\n\nThe data type defined for the queue allows for a string for event name, time, variant data type for longer descriptors or data and the stop condition but this can be expanded to allow for any number of variables to be written.\n\nWith each call to Add, an event is added to the Queue that needs to be read off and written.  The HypervisorWrite.vi is called in a parallel loop below to log these events as they are added to the queue."
  # "Copyright © 2017 Epimedia, Inc. All Rights Reserved.\n\nThe Epimedia Application Library is Copyright © 2009-2017 Epimedia, Inc. \nAll Rights Reserved. Used under license."
